vi "VSSDecodeFIRASimBall.vi"(8 "error in (no error)":errorcluster, 9 "TimeStamp":timestamp, 11 "Frame":u8[](array[numeric])) -> (0 "error out":errorcluster, 2 "Robots":u8[](array[numeric]), 3 "Balls out":T1[](array[typedef]))   [LabVIEW 2023]
uses:
  Controls/SSL Detection Ball.ctl
  <vilib>/Analysis/Matrix/Datatypes/RealMatrix.ctl
  <vilib>/Analysis/Matrix/NI_Matrix.lvlib
panel:
  in  "Ball":T1
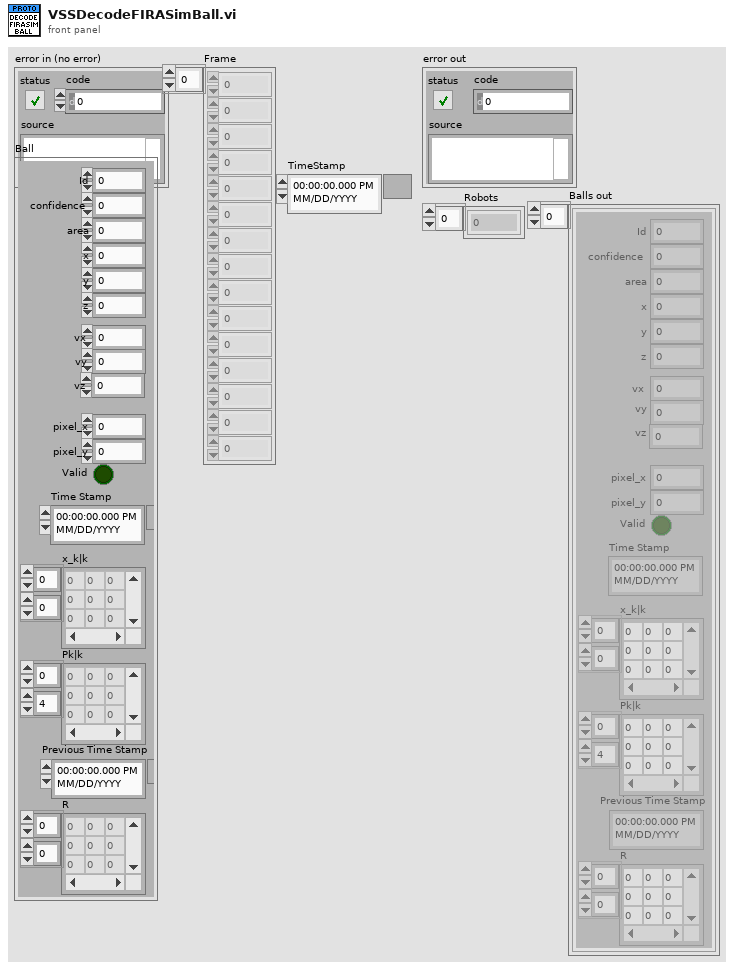
[diagram p1: front panel]
types:
  T1 = typedef "SSL Detection Ball.ctl" = cluster{"x":sgl, "area":u32, "confidence":sgl, "y":sgl, "z":sgl, "pixel_x":sgl, "pixel_y":sgl, "Valid":bool, "Time Stamp":timestamp, "x_k|k":T2, "Pk|k":T2, "Id":u32, "Previous Time Stamp":timestamp, "R":T2, " vx":sgl, "vy":dbl, "vz":dbl}
  T2 = typedef "NI_Matrix.lvlib/RealMatrix.ctl" = dbl[][]
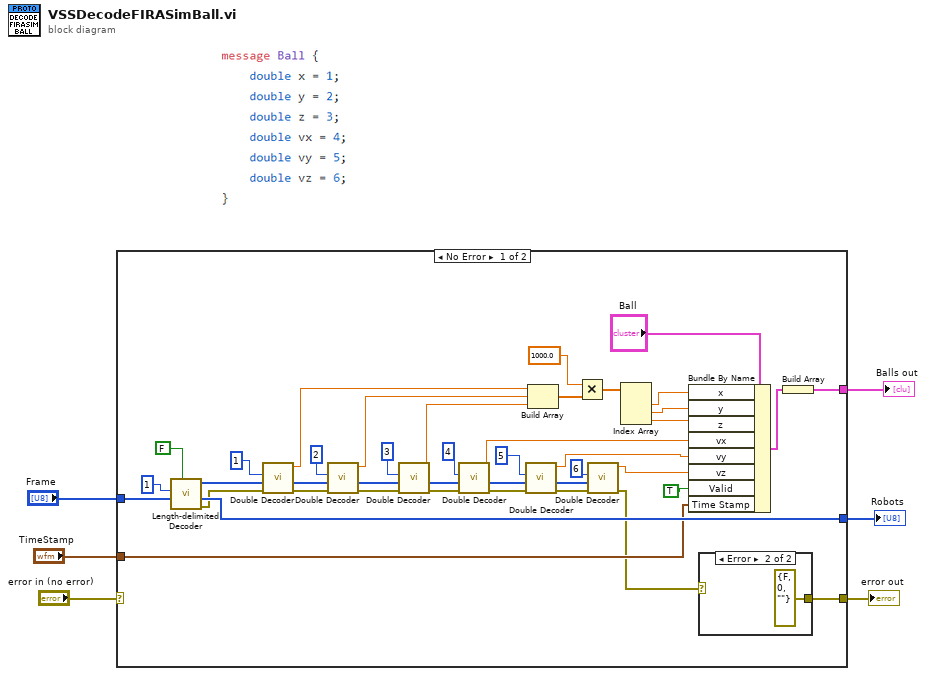
[diagram p0: block diagram]
diagram:
  n1 = case shown="No Error" "error in (no error)" {
    selector: "error in (no error)" -> [_ w50]
    tunnel: [w7 w50] -> w5
    tunnel: "Frame" -> [w47 _]
    tunnel: [w45 _] -> w3
    tunnel: [w31 _] -> w1
    tunnel: "TimeStamp" -> [w32 _]
    frame No Error {
      n2 = call "Length-delimited Decoder.vi"("Optional"=FALSE, "Array"=w47, "Key"=1) -> ("error out"=w35:errorcluster, "array w/ subset deleted"=w45:u8[], "Length-delimited"=w44:u8[])  [unwired: 5 in, 1 out]
      n3 = call "Double Decoder.vi"("error in (no error)"=w35, "Array"=w44, "Key"=1) -> ("error out"=w36:errorcluster, "array w/ subset deleted"=w43:u8[], "Double"=w29:dbl)  [unwired: 5 in, 1 out]
      n4 = call "Double Decoder.vi"("error in (no error)"=w36, "Array"=w43, "Key"=2) -> ("error out"=w34:errorcluster, "array w/ subset deleted"=w42:u8[], "Double"=w28:dbl)  [unwired: 5 in, 1 out]
      n5 = call "Double Decoder.vi"("error in (no error)"=w34, "Array"=w42, "Key"=3) -> ("error out"=w33:errorcluster, "array w/ subset deleted"=w16:u8[], "Double"=w27:dbl)  [unwired: 5 in, 1 out]
      n6 = call "Double Decoder.vi"("error in (no error)"=w33, "Array"=w16, "Key"=4) -> ("error out"=w10:errorcluster, "array w/ subset deleted"=w15:u8[], "Double"=w20:dbl)  [unwired: 5 in, 1 out]
      n7 = call "Double Decoder.vi"("error in (no error)"=w10, "Array"=w15, "Key"=5) -> ("error out"=w9:errorcluster, "array w/ subset deleted"=w14:u8[], "Double"=w19:dbl)  [unwired: 5 in, 1 out]
      n8 = Build Array(w29, w28, w27) -> (w26:dbl[])
      n9 = Multiply(x=1000.0, y=w26) -> (x*y=w24:dbl[])
      n10 = call "Double Decoder.vi"("error in (no error)"=w9, "Array"=w14, "Key"=6) -> ("error out"=w8:errorcluster, "Double"=w18:dbl)  [unwired: 5 in, 2 out]
      n11 = Index Array(array=w24) -> (element #1=w23:dbl, element #2=w22:dbl, element #3=w21:dbl)  [unwired: 3 in]
      n12 = Bundle By Name(cluster="Ball", "x"=w23, "y"=w22, "z"=w21, "vx"=w20, "vy"=w19, "vz"=w18, "Valid"=TRUE, "Time Stamp"=w32) -> (w30:T1)
      n13 = case shown="Error" w8 {
        selector: w8 -> [w48 _]
        tunnel: [w48 errorcluster {"status"=FALSE, "code"=0, "source"=""} ("error IO")] -> w7
        frame No Error {
        }
        frame Error {
        }
      }
      n14 = Build Array(w30) -> (w31:T1[])
    }
    frame Error {
    }
  }
  "error out" <- w5
  "Robots" <- w3
  "Balls out" <- w1
